vi "41_42_UNDT_Encoder1CurrData (SubVI).vi"(8 "error in":errorcluster, 10 "Encoder1CurrData":i64, 11 "String in":refnum<vi>) -> (0 "error out":errorcluster)   [LabVIEW 2017]
uses:
  Global_SNK3_HF.vi
  LV_Unicorn/LV_Unicorn.lvlib
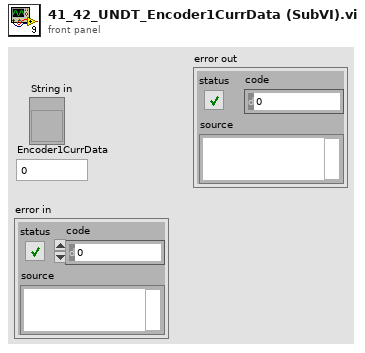
[diagram p1: front panel]
types:
  T1 = typedef "LV_Unicorn.lvlib/unicorn_Param.ctl" = cluster{"conParam":T2, "Param":T3}
  T2 = typedef "LV_Unicorn.lvlib/unicorn_conn.ctl" = cluster{"ReadIntParam":bool, "ReadDescrParam":bool, "ReadFloatParam":bool, "debug":bool, "ReadJSON":bool, "IP_address":string, "N_attempts":i32, "type_con":enum16{"Serial", "TCP"}, "MB_address":i32, "VISA":refnum<visa-resource-name>, "connection ID":refnum<k5>, "nameDevices":string, "timeout":i32, "port":u16, "type_version":string, "baud_rate":u32, "VersionControl":bool, "TCP_conn":bool, "WindowSize":i32}
  T3 = typedef "LV_Unicorn.lvlib/unicorn_JSON.ctl" = cluster{"NumParam":cluster{"NTelem":i32, "NInt":i32, "NFloat":i32, "NTable":i32}, "ParamInt":T4, "Telemetry":T5, "Table":T6, "ParamFloat":T7}
  T4 = typedef "LV_Unicorn.lvlib/unicorn_ParamInt.ctl" = cluster{"ID":string, "Num":i32, "Name":string, "Type":string, "Enum":string, "Desc":string, "Unit":string, "Access":string, "FormatStr":string, "Min":i32, "Max":i32}[]
  T5 = typedef "LV_Unicorn.lvlib/unicorn_Telemetry.ctl" = cluster{"ID":string, "Num":i32, "Name":string, "Desc":string, "Unit":string, "FormatStr":string, "Min":i32, "Max":i32}[]
  T6 = typedef "LV_Unicorn.lvlib/unicorn_Table.ctl" = cluster{"Num":i32, "Access":string, "ColumnCount":i32, "NeedParamPrepare":bool, "Columns":cluster{"Column":i32, "Desc":string, "Name":string}[], "DataType":string, "FormatStr":string, "ID":string, "Name":string, "RowCount":i32, "Rows":cluster{"Desc":string, "ID":string, "Max":i32, "Min":i32, "Name":string, "Row":i32, "Unit":string}[], "Type":string}[]
  T7 = typedef "LV_Unicorn.lvlib/unicorn_ParamFloat.ctl" = cluster{"ID":string, "Num":i32, "Name":string, "Type":string, "Enum":string, "Desc":string, "Unit":string, "Access":string, "FormatStr":string, "Min":sgl, "Max":sgl}[]
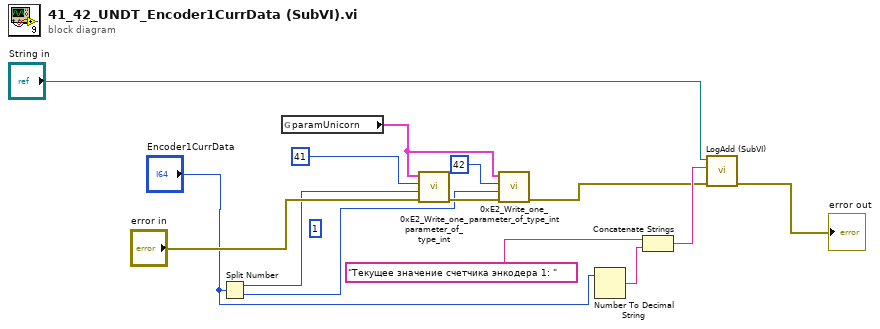
[diagram p0: block diagram]
diagram:
  (unwired) 1 ("Номер параметра")
  n1 = Split Number(x="Encoder1CurrData") -> (hi(x)=w8:u32, lo(x)=w6:u32)
  n2 = global read "Global_SNK3_HF.vi" "paramUnicorn"() -> (w4:T1)
  n3 = call "0xE2_Write_one_parameter_of_type_int.vi"("error in"="error in", "ParamIn"=w8, "NumParamIn"=41 ("Номер параметра"), "paramUnicorn 2"=w4) -> ("error out"=w7:errorcluster)  [unwired: 4 in, 3 out]
  n4 = call "0xE2_Write_one_parameter_of_type_int.vi"("error in"=w7, "ParamIn"=w6, "NumParamIn"=42 ("Номер параметра"), "paramUnicorn 2"=w4) -> ("error out"=w3:errorcluster)  [unwired: 4 in, 3 out]
  n5 = Number To Decimal String(number="Encoder1CurrData") -> (decimal integer string=w1:string)  [unwired: 1 in]
  n6 = Concatenate Strings("Текущее значение счетчика энкодера 1: " ("string"), w1) -> (w10:string)
  n7 = call "LogAdd (SubVI).vi"("error in"=w3, "string"=w10, "Log"="String in") -> ("error out"=→"error out":errorcluster)  [unwired: 8 in]
